vi "TIO Data Stream Receiver.vi"(9 "Stream Info In":T1(array[cluster]) {"Timestamp type" format="%x"; "Flags" format="%x"; "Data Type" items=["INT8"=16, "UINT8"=17, "UINT16"=32, "INT16"=33, "UINT24"=48, "INT24"=49, "UINT32"=64, "INT32"=65, "UINT64"=128, "INT64"=129, "FLOAT32"=66, "FLOAT64"=130]}, 10 "Raw Stream Data":string, 11 "Stream ID":u16) -> (0 "Known Stream":bool, 1 "Stream Info Out":T1(array[cluster]) {"Timestamp type" format="%x"; "Flags" format="%x"; "Data Type" items=["INT8"=16, "UINT8"=17, "UINT16"=32, "INT16"=33, "UINT24"=48, "INT24"=49, "UINT32"=64, "INT32"=65, "UINT64"=128, "INT64"=129, "FLOAT32"=66, "FLOAT64"=130]}, 3 "Data Stream Notification":T2={"Stream Description"={"Stream ID"=0, "Data Type"=66, "Channels"=3, "Restart ID"=0, "Start timestamp (s)"=0.20090000000000002, "Sample counter"=382825, "Period (s)"=0.005, "Flags"=1, "Timestamp type"=1, "Name"="gmr.cal", "Last sample number"=0, "Last Restart ID"=0, "Version"=0, "Sample Size"=0}, "Sample #"=0, "Raw Data"=""} {"Stream Description"."Timestamp type" format="%x"; "Stream Description"."Flags" format="%x"; "Stream Description"."Data Type" items=["INT8"=16, "UINT8"=17, "UINT16"=32, "INT16"=33, "UINT24"=48, "INT24"=49, "UINT32"=64, "INT32"=65, "UINT64"=128, "INT64"=129, "FLOAT32"=66, "FLOAT64"=130]})   [LabVIEW 2017]
panel:
  # "TODO: Implement sample number rollover"
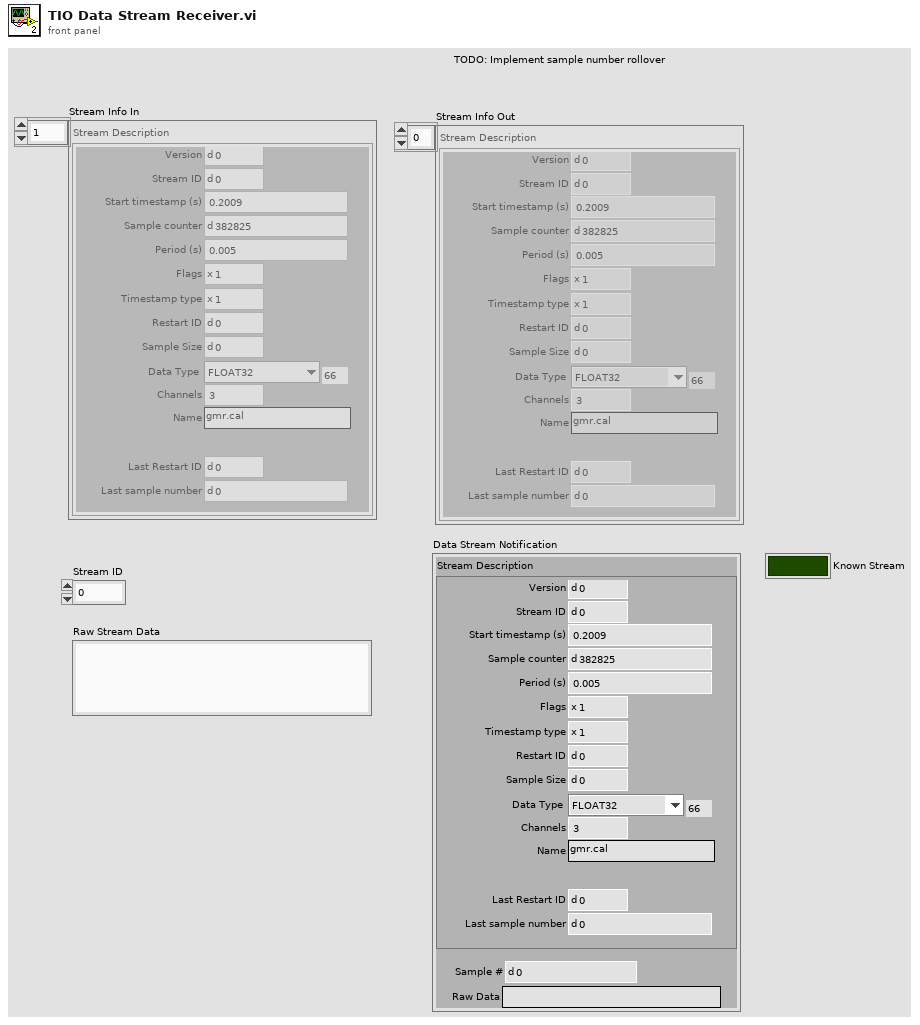
[diagram p1: front panel]
types:
  T1 = cluster{"Stream ID":u16, "Data Type":u8, "Channels":u8, "Restart ID":u16, "Start timestamp (s)":dbl, "Sample counter":u64, "Period (s)":dbl, "Flags":u8, "Timestamp type":u8, "Name":string, "Last sample number":u64, "Last Restart ID":u16, "Version":u16, "Sample Size":u16}[]
  T2 = cluster{"Stream Description":cluster{"Stream ID":u16, "Data Type":u8, "Channels":u8, "Restart ID":u16, "Start timestamp (s)":dbl, "Sample counter":u64, "Period (s)":dbl, "Flags":u8, "Timestamp type":u8, "Name":string, "Last sample number":u64, "Last Restart ID":u16, "Version":u16, "Sample Size":u16}, "Sample #":u32, "Raw Data":string}
  T3 = cluster{"Stream ID":u16, "Data Type":u8, "Channels":u8, "Restart ID":u16, "Start timestamp (s)":dbl, "Sample counter":u64, "Period (s)":dbl, "Flags":u8, "Timestamp type":u8, "Name":string, "Last sample number":u64, "Last Restart ID":u16, "Version":u16, "Sample Size":u16}
  T4 = cluster{"Stream Description":cluster{"Stream ID":u16, "Data Type":u8, "Channels":u8, "Restart ID":u16, "Start timestamp (s)":dbl, "Sample counter":u64, "Period (s)":dbl, "Flags":u8, "Timestamp type":u8, "Name":string, "Last sample number":u64, "Last Restart ID":u16, "Version":u16, "Sample Size":u16}, "U32":u32, "Raw Stream Data":string}
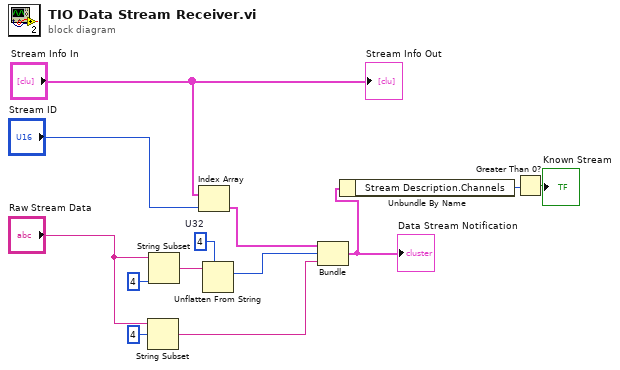
[diagram p0: block diagram]
diagram:
  w6 = u32 4  # U32
  n1 = String Subset(string="Raw Stream Data", offset (0)=4) -> (substring=w11:string)  [unwired: 1 in]
  n2 = String Subset(string="Raw Stream Data", length (rest)=4 ("offset (0)")) -> (substring=w5:string)  [unwired: 1 in]
  n3 = Index Array(array="Stream Info In", index="Stream ID") -> (element=w12:T3)
  n4 = Unflatten From String(type=w6, binary string=w5) -> (value=w4:u32)  [unwired: 3 in, 2 out]
  n5 = Bundle("Stream Description"=w12, "U32"=w4, "Raw Stream Data"=w11) -> (w3:T4)  [unwired: 1 in]
  "Data Stream Notification" <- w3
  n6 = Unbundle By Name(w3) -> ("Stream Description.Channels"=w2:u8)
  n7 = Greater Than 0?(x=w2) -> (x > 0?=→"Known Stream":bool)
  "Stream Info Out" <- "Stream Info In"
